vi "PFI-28000-System_Create.vi"(0 "Address":string, 5 "Port":u16, 11 "error in (no error)":errorcluster) -> (4 "PFI-28000-System out":refnum<class "PFI-28000-System.lvclass">, 15 "error out":errorcluster)   [LabVIEW 2017, in "PFI-28000-System.lvclass"]
uses:
  PFI-28000-System.lvclass
  C:/wc/07143 Precision Filters 28000 Support/Driver/source/Base/PFI-28000-Base.lvclass
  Overload/PFI-28000-Overload.lvclass
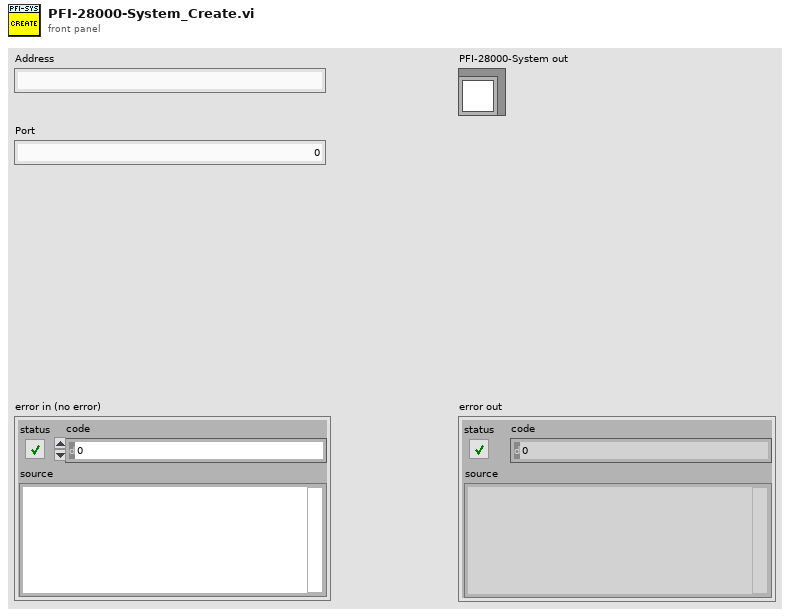
[diagram p1: front panel]
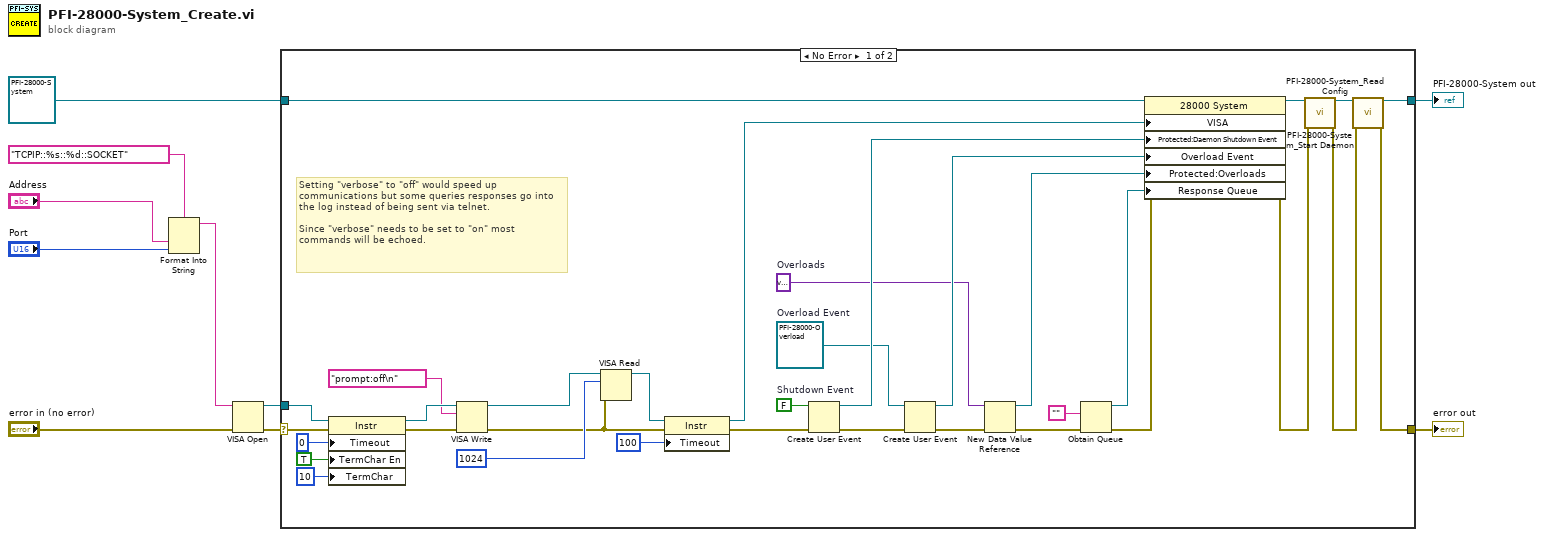
[diagram p0: block diagram]
diagram:
  n1 = Format Into String(format string="TCPIP::%s::%d::SOCKET" ("empty string"), "Address", "Port") -> (resulting string=w4:string)  [unwired: 2 in, 1 out]
  n2 = VISA Open(error in (no error)="error in (no error)", VISA resource name=w4) -> (VISA resource name=w6:refnum<visa-resource-name>, error out=w7:errorcluster)  [unwired: 3 in]
  n3 = case shown="No Error" w7 {
    selector: w7 -> [w44 w45]
    tunnel: w6 -> [w43 _]
    tunnel: refnum<class "PFI-28000-System.lvclass"> refnum ("PFI-28000-System out") -> [w40 w46]
    tunnel: [w26 w45] -> w2
    tunnel: [w25 w46] -> w1
    frame No Error {
      w20 = variant  # Overloads
      w34 = refnum<class "PFI-28000-Overload.lvclass"> refnum  # Overload Event
      w38 = FALSE  # Shutdown Event
      # "Setting \"verbose\" to \"off\" would speed up communications but some queries responses go into the log instead of being sent via telnet.\n\nSince \"verbose\" needs to be set to \"on\" most commands will be echoed."
      n4 = property class="Instr"(reference=w43, error in=w44, "Timeout"=u32 0 ("General Settings:Timeout Value"), "TermChar En"=TRUE ("Message Based Settings:Termination Character Enable"), "TermChar"=u8 10 ("Message Based Settings:Termination Character")) -> (reference out=w24:refnum<visa-resource-name>, error out=w39:errorcluster)
      n5 = VISA Write(VISA resource name=w24, write buffer="prompt:off\n" ("empty string"), error in (no error)=w39) -> (VISA resource name out=w12:refnum<visa-resource-name>, error out=w11:errorcluster)  [unwired: 1 out]
      n6 = VISA Read(VISA resource name=w12, byte count=u32 1024, error in (no error)=w11) -> (VISA resource name out=w16:refnum<visa-resource-name>)  [unwired: 3 out]
      n7 = property class="Instr"(reference=w16, error in=w11, "Timeout"=u32 100 ("General Settings:Timeout Value")) -> (reference out=w13:refnum<visa-resource-name>, error out=w15:errorcluster)
      n8 = Create User Event(user event datatype=w38, error in=w15) -> (user event=w36:refnum<user-event>, error out=w37:errorcluster)
      n9 = Create User Event(user event datatype=w34, error in=w37) -> (user event=w35:refnum<user-event>, error out=w22:errorcluster)
      n10 = New Data Value Reference(data value=w20, error in=w22) -> (data value reference=w19:refnum<data-value>, error out=w21:errorcluster)
      n11 = Obtain Queue(element data type="", error in (no error)=w21) -> (queue out=w32:refnum<queue>, error out=w31:errorcluster)  [unwired: 3 in, 1 out]
      n12 = property class="28000 System"(reference=w40, error in=w31, "VISA"=w13, "Protected:Daemon Shutdown Event"=w36, "Overload Event"=w35, "Protected:Overloads"=w19, "Response Queue"=w32) -> (reference out=w30:refnum<class "PFI-28000-System.lvclass">, error out=w29:errorcluster)
      n13 = call "PFI-28000-System_Start Daemon.vi"("PFI-28000-System in"=w30, "error in (no error)"=w29) -> ("PFI-28000-System out"=w28:refnum<class "PFI-28000-System.lvclass">, "error out"=w27:errorcluster)  [unwired: 12 in]
      n14 = call "PFI-28000-System_Read Config.vi"("PFI-28000-System in"=w28, "error in (no error)"=w27) -> ("PFI-28000-System out"=w25:refnum<class "PFI-28000-System.lvclass">, "error out"=w26:errorcluster)  [unwired: 12 in]
    }
    frame Error {
    }
  }
  "error out" <- w2
  "PFI-28000-System out" <- w1
